vi "str_to_BSON_bytes.vi"(11 "value":string) -> (3 "BSONbytes":u8[](array[numeric]) format="%02d")   [LabVIEW 2015, in "BSON_convertors_Library.lvlib"]
uses:
  BSON_convertors_Library.lvlib
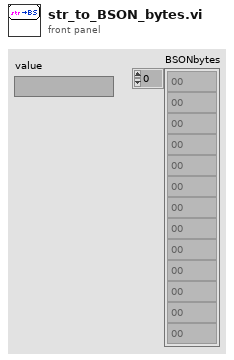
[diagram p1: front panel]
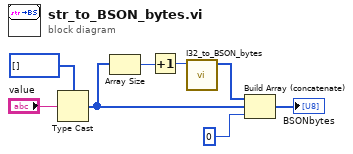
[diagram p0: block diagram]
diagram:
  n1 = Type Cast(type=u8[] [] ("*(type *) &x"), x="value") -> (*(type *) &x=w3:u8[])
  n2 = Array Size(array=w3) -> (size(s)=w6:i32)
  n3 = Increment(x=w6) -> (x+1=w5:i32)
  n4 = call "I32_to_BSON_bytes.vi"("value"=w5) -> ("BSONbytes"=w4:u8[])  [unwired: 10 in]
  n5 = Build Array (concatenate)(w4, w3, u8 0) -> (→"BSONbytes":u8[])
